vi "LG DIAdem Run Report Generation Script.vi"(0 "Data Source File Path (*.tdms)":path, 5 "DIAdem Report Template File Path (*.tdr)":path, 7 "Report File Path (*.png)":path, 9 "Script File Path (*.vbs)":path, 11 "error in (no error)":errorcluster) -> (15 "error out":errorcluster)   [LabVIEW 2018, in "LG_DIAdemAutomation.lvlib"]
uses:
  LG_DIAdemAutomation.lvlib
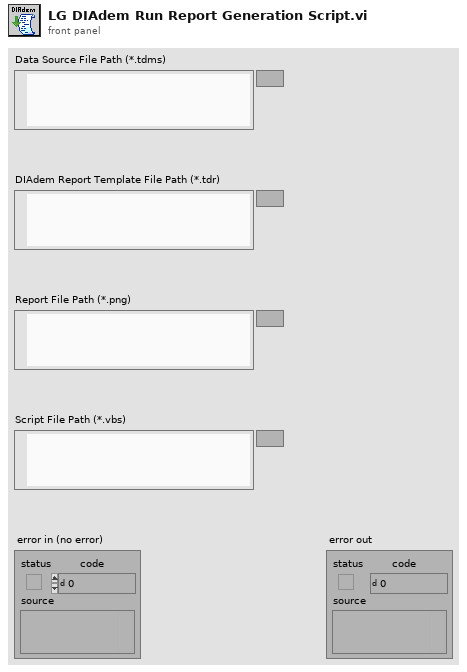
[diagram p1: front panel]
types:
  T1 = typedef "DIAdem Reference.ctl" = cluster{"ToCommand Reference":refnum<k7>, "ToDataSheet Reference":refnum<k7>}
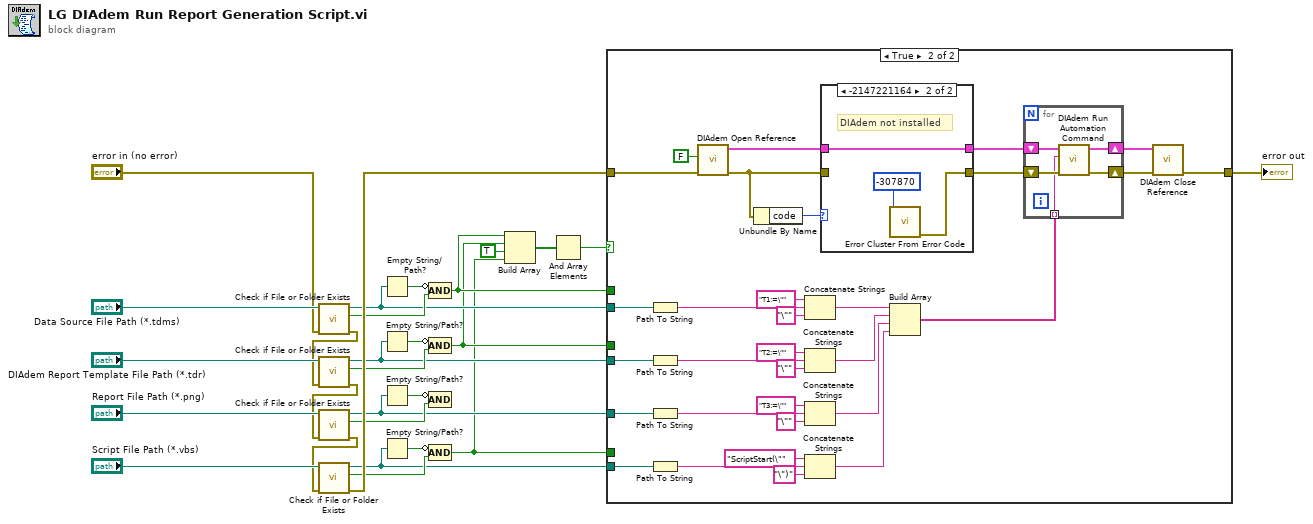
[diagram p0: block diagram]
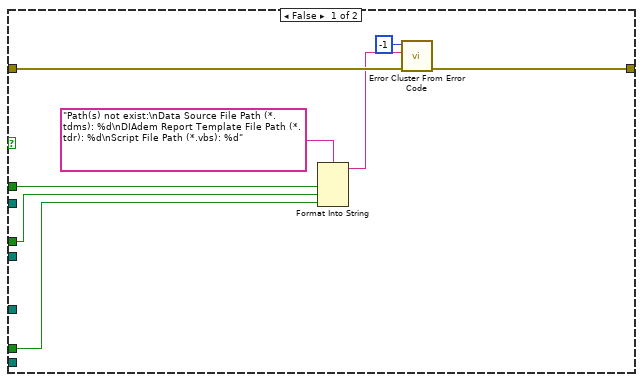
[diagram p2: hidden frame]
diagram:
  n1 = call <vilib>:"Check if File or Folder Exists.vi"("error in (no error)"="error in (no error)", "path"="Data Source File Path (*.tdms)") -> ("error out"=w22:errorcluster, "file or folder exists?"=w15:bool, "dup path"=w5:path)  [unwired: 7 in]
  n2 = call <vilib>:"Check if File or Folder Exists.vi"("error in (no error)"=w22, "path"="DIAdem Report Template File Path (*.tdr)") -> ("error out"=w21:errorcluster, "file or folder exists?"=w9:bool, "dup path"=w8:path)  [unwired: 7 in]
  n3 = call <vilib>:"Check if File or Folder Exists.vi"("error in (no error)"=w21, "path"="Report File Path (*.png)") -> ("error out"=w20:errorcluster, "file or folder exists?"=w10:bool, "dup path"=w7:path)  [unwired: 7 in]
  n4 = call <vilib>:"Check if File or Folder Exists.vi"("error in (no error)"=w20, "path"="Script File Path (*.vbs)") -> ("error out"=w19:errorcluster, "file or folder exists?"=w11:bool, "dup path"=w6:path)  [unwired: 7 in]
  n5 = Empty String/Path?(string/path=w5) -> (empty?=w16:bool)
  n6 = Empty String/Path?(string/path=w8) -> (empty?=w14:bool)
  n7 = Empty String/Path?(string/path=w7) -> (empty?=w13:bool)
  n8 = Empty String/Path?(string/path=w6) -> (empty?=w12:bool)
  n9 = Compound Arithmetic op=AND(invert w16, w15) -> (w4:bool)
  n10 = Compound Arithmetic op=AND(invert w14, w9) -> (w3:bool)
  n11 = Compound Arithmetic op=AND(invert w13, w10) -> ()  [unwired: 1 out]
  n12 = Compound Arithmetic op=AND(invert w12, w11) -> (w2:bool)
  n13 = Build Array(w4, w3, TRUE ("element"), w2) -> (w18:bool[])
  n14 = And Array Elements(Boolean array=w18) -> (logical AND=w17:bool)
  n15 = case shown="True" w17 {
    tunnel: [w35 w67] -> w28
    tunnel: w5 -> [_ w50]
    tunnel: w8 -> [_ w49]
    tunnel: w7 -> [_ w48]
    tunnel: w6 -> [_ w47]
    tunnel: w19 -> [w36 w46]
    tunnel: w4 -> [w32 _]
    tunnel: w3 -> [w31 _]
    tunnel: w2 -> [w30 _]
    frame False {
      n16 = Format Into String(format string="Path(s) not exist:\nData Source File Path (*.tdms): %d\nDIAdem Report Template File Path (*.tdr): %d\nScript File Path (*.vbs): %d" ("error message (\"\")"), w32, w31, w30) -> (resulting string=w34:string)  [unwired: 2 in, 1 out]
      n17 = call <vilib>:"Error Cluster From Error Code.vi"("error in (no error)"=w36, "error message (\"\")"=w34, "error code (0)"=-1) -> ("error out"=w35:errorcluster)  [unwired: 6 in]
    }
    frame True {
      n18 = Path To String(path=w50) -> (string=w65:string)
      n19 = Path To String(path=w49) -> (string=w62:string)
      n20 = Path To String(path=w48) -> (string=w59:string)
      n21 = Path To String(path=w47) -> (string=w56:string)
      n22 = call <vilib>:"DIAdem Open Reference.vi"("error in (no error)"=w46, "Show Environment (F)"=FALSE) -> ("error out"=w41:errorcluster, "DIAdem Reference"=w42:T1)  [unwired: 8 in]
      n23 = Unbundle By Name(w41) -> ("code"=w43:i32)
      n24 = Concatenate Strings("T1:=\"" ("string"), w65, "\"" ("string")) -> (w54:string)
      n25 = Concatenate Strings("T2:=\"" ("string"), w62, "\"" ("string")) -> (w51:string)
      n26 = Concatenate Strings("T3:=\"" ("string"), w59, "\"" ("string")) -> (w52:string)
      n27 = Concatenate Strings("ScriptStart(\"" ("string"), w56, "\")" ("string")) -> (w53:string)
      n28 = case shown="-2147221164" w43 {
        tunnel: [w74 w76] -> w40
        tunnel: w41 -> [w74 _]
        tunnel: [w73 w77] -> w39
        tunnel: w42 -> [w73 w77]
        frame 0, Default {
        }
        frame -2147221164 {
          # "DIAdem not installed"
          n29 = call <vilib>:"Error Cluster From Error Code.vi"("error code (0)"=-307870 ("Code")) -> ("error out"=w76:errorcluster)  [unwired: 8 in]
        }
      }
      n30 = Build Array(w54, w51, w52, w53) -> (w45:string[])
      n31 = for {
        shift-right: [w69] -> w37
        shift-left: w40 -> [w72]
        shift-right: [w70] -> w38
        shift-left: w39 -> [w71]
        tunnel: w45 -> [w68] mode=indexing
        n32 = call <vilib>:"DIAdem Run Automation Command.vi"("error in (no error)"=w72, "command"=w68, "DIAdem Reference"=w71) -> ("error out"=w69:errorcluster, "DIAdem Reference"=w70:T1)  [unwired: 7 in]
      }
      n33 = call <vilib>:"DIAdem Close Reference.vi"("error in (no error)"=w37, "DIAdem Reference"=w38) -> ("error out"=w67:errorcluster)  [unwired: 9 in]
    }
  }
  "error out" <- w28
